vi "Speed Math.vi"(2 "Throttle":dbl, 3 "Twist":dbl) -> (0 "Right Wheel Velocity":dbl, 1 "Left Wheel Velocity":dbl)   [LabVIEW 2017]
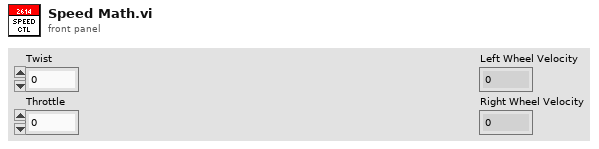
[diagram p1: front panel]
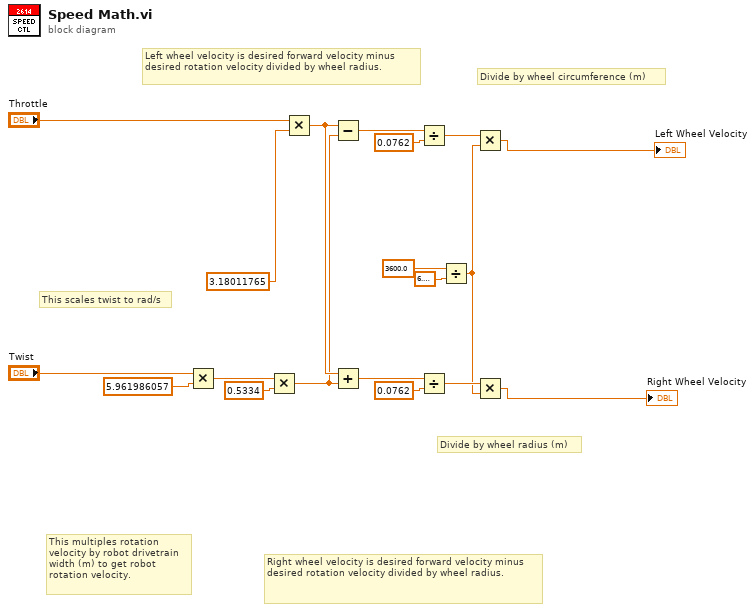
[diagram p0: block diagram]
diagram:
  # "Divide by wheel circumference (m)"
  # "Divide by wheel radius (m)"
  # "Right wheel velocity is desired forward velocity minus desired rotation velocity divided by wheel radius."
  # "This multiples rotation velocity by robot drivetrain width (m) to get robot rotation velocity."
  # "Left wheel velocity is desired forward velocity minus desired rotation velocity divided by wheel radius."
  # "This scales twist to rad/s"
  n1 = Multiply(x="Twist", y=5.961986057) -> (x*y=w17:dbl)
  n2 = Multiply(x=w17, y=0.5334) -> (x*y=w14:dbl)
  n3 = Multiply(x="Throttle", y=3.18011765) -> (x*y=w15:dbl)
  n4 = Subtract(x=w15, y=w14) -> (x-y=w12:dbl)
  n5 = Add(x=w15, y=w14) -> (x+y=w13:dbl)
  n6 = Divide(x=w12, y=0.0762) -> (x/y=w9:dbl)
  n7 = Divide(x=w13, y=0.0762) -> (x/y=w8:dbl)
  n8 = Divide(x=3600.0, y=6.283185307179586) -> (x/y=w4:dbl)
  n9 = Multiply(x=w9, y=w4) -> (x*y=→"Left Wheel Velocity":dbl)
  n10 = Multiply(x=w8, y=w4) -> (x*y=→"Right Wheel Velocity":dbl)
